vi "PI_Controller.vi"(0 "error":sgl format="%#_13g", 1 "reset? (F)":bool, 2 "Resources":T1, 5 "enable bumpless transfer? (F)":bool, 7 "manual control":T6, 11 "state in":T3, 12 "gains":T4 {"proportional gain" step=0.125}, 13 "output range":T5={"output high (Inf)"=inf, "output low (-Inf)"=-inf}) -> (4 "output":sgl, 6 "error":sgl, 8 "actions":T2, 15 "state out":T3)   [LabVIEW 2017]
uses:
  <vilib>/rvi/Analysis/control/PID/Typedef/niFpgaPID_ManualControl.ctl
  <vilib>/rvi/Analysis/control/PID/Typedef/niFpgaPID_OutputRange.ctl
  <vilib>/rvi/Analysis/control/PID/Typedef/niFpgaPID_PIGains.ctl
  <vilib>/rvi/Analysis/control/PID/Typedef/niFpgaPID_PIState.ctl
  <vilib>/rvi/Analysis/control/PID/Typedef/niFpgaPID_PIActions.ctl
  Multiplier/Multiplier.lvclass
  Adder/Adder.lvclass
  Subtractor/Subtractor.lvclass
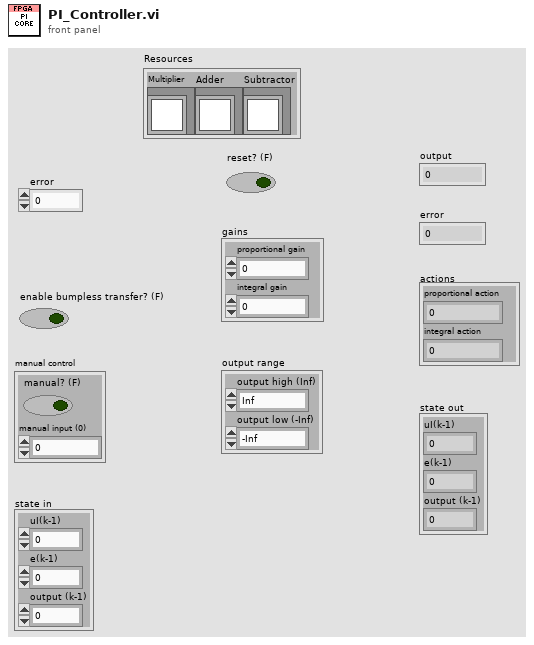
[diagram p1: front panel]
types:
  T1 = cluster{"Multiplier":refnum<class "Multiplier.lvclass">, "Adder":refnum<class "Adder.lvclass">, "Subtractor":refnum<class "Subtractor.lvclass">}
  T2 = typedef "niFpgaPID_PIActions.ctl" = cluster{"proportional action":sgl, "integral action":sgl}
  T3 = typedef "niFpgaPID_PIState.ctl" = cluster{"uI(k-1)":sgl, "e(k-1)":sgl, "output (k-1)":sgl}
  T4 = typedef "niFpgaPID_PIGains.ctl" = cluster{"proportional gain":sgl, "integral gain":sgl}
  T5 = typedef "niFpgaPID_OutputRange.ctl" = cluster{"output high (Inf)":sgl, "output low (-Inf)":sgl}
  T6 = typedef "niFpgaPID_ManualControl.ctl" = cluster{"manual? (F)":bool, "manual input (0)":sgl}
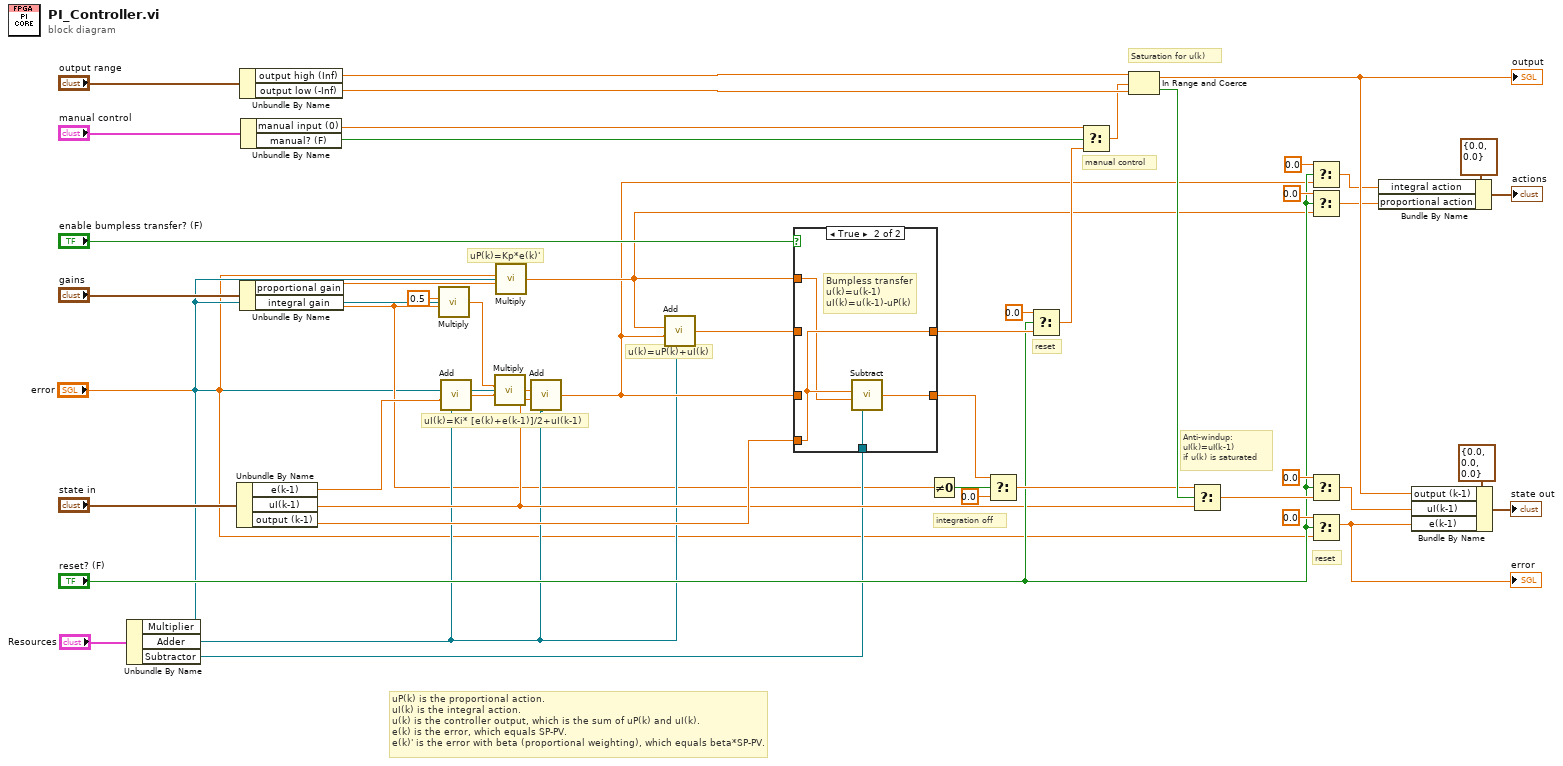
[diagram p0: block diagram]
diagram:
  # "uP(k) is the proportional action.\nuI(k) is the integral action.\nu(k) is the controller output, which is the sum of uP(k) and uI(k).\ne(k) is the error, which equals SP-PV.\ne(k)' is the error with beta (proportional weighting), which equals beta*SP-PV."
  # "integration off"
  # "reset"
  # "manual control"
  # "reset"
  # "Anti-windup:\nuI(k)=uI(k-1) \nif u(k) is saturated"
  # "Saturation for u(k)"
  # "u(k)=uP(k)+uI(k)"
  # "uI(k)=Ki* [e(k)+e(k-1)]/2+uI(k-1)"
  # "uP(k)=Kp*e(k)'"
  n1 = Unbundle By Name("Resources") -> ("Multiplier"=w2:refnum<class "Multiplier.lvclass">, "Adder"=w7:refnum<class "Adder.lvclass">, "Subtractor"=w6:refnum<class "Subtractor.lvclass">)
  n2 = Unbundle By Name("state in") -> ("e(k-1)"=w15:sgl, "uI(k-1)"=w14:sgl, "output (k-1)"=w43:sgl)
  n3 = Unbundle By Name("output range") -> ("output high (Inf)"=w31:sgl, "output low (-Inf)"=w30:sgl)
  n4 = Unbundle By Name("gains") -> ("proportional gain"=w11:sgl, "integral gain"=w4:sgl)
  n5 = Unbundle By Name("manual control") -> ("manual input (0)"=w40:sgl, "manual? (F)"=w39:bool)
  n6 = call-dynamic "Multiply.vi"("x"=sgl 0.5, "y"=w4, "Multiplier"=w2) -> ("x*y"=w5:sgl)  [unwired: 4 in]
  n7 = call-dynamic "Add.vi"("x"="error", "y"=w15, "Adder"=w7) -> ("x+y"=w13:sgl)  [unwired: 4 in]
  n8 = call-dynamic "Multiply.vi"("x"=w5, "y"=w13, "Multiplier"=w2) -> ("x*y"=w12:sgl)  [unwired: 4 in]
  n9 = call-dynamic "Multiply.vi"("x"="error", "y"=w11, "Multiplier"=w2) -> ("x*y"=w10:sgl)  [unwired: 4 in]
  n10 = call-dynamic "Add.vi"("x"=w12, "y"=w14, "Adder"=w7) -> ("x+y"=w9:sgl)  [unwired: 4 in]
  n11 = call-dynamic "Add.vi"("x"=w10, "y"=w9, "Adder"=w7) -> ("x+y"=w8:sgl)  [unwired: 4 in]
  n12 = case shown="True" "enable bumpless transfer? (F)" {
    tunnel: w8 -> [w52 _]
    tunnel: [w52 w56] -> w36
    tunnel: w9 -> [w51 _]
    tunnel: [w51 w54] -> w38
    tunnel: w10 -> [_ w55]
    tunnel: w43 -> [_ w56]
    tunnel: w6 -> [_ w53]
    frame False {
    }
    frame True {
      # "Bumpless transfer\nu(k)=u(k-1)\nuI(k)=u(k-1)-uP(k)"
      n13 = call-dynamic "Subtract.vi"("x"=w56, "y"=w55, "Subtractor"=w53) -> ("x-y"=w54:sgl)  [unwired: 4 in]
    }
  }
  n14 = Not Equal To 0?(x=w4) -> (x != 0?=w42:bool)
  n15 = Select(t=w38, s=w42, f=sgl 0.0) -> (s? t:f=w20:sgl)
  n16 = Select(t=sgl 0.0 ("f"), s="reset? (F)", f=w36) -> (s? t:f=w35:sgl)
  n17 = Select(t=w40, s=w39, f=w35) -> (s? t:f=w29:sgl)
  n18 = In Range and Coerce(upper limit=w31, x=w29, lower limit=w30) -> (coerced(x)=w28:sgl, In Range?=w32:bool)
  "output" <- w28
  n19 = Select(t=w20, s=w32, f=w14) -> (s? t:f=w21:sgl)
  n20 = Select(t=sgl 0.0, s="reset? (F)", f=w9) -> (s? t:f=w24:sgl)
  n21 = Select(t=sgl 0.0, s="reset? (F)", f=w10) -> (s? t:f=w25:sgl)
  n22 = Select(t=sgl 0.0, s="reset? (F)", f=w21) -> (s? t:f=w19:sgl)
  n23 = Select(t=sgl 0.0, s="reset? (F)", f="error") -> (s? t:f=w17:sgl)
  "error" <- w17
  n24 = Bundle By Name(cluster=T2 {"proportional action"=0.0, "integral action"=0.0} ("actions"), "integral action"=w24, "proportional action"=w25) -> (→"actions":T2)
  n25 = Bundle By Name(cluster=T3 {"uI(k-1)"=0.0, "e(k-1)"=0.0, "output (k-1)"=0.0} ("state out"), "output (k-1)"=w28, "uI(k-1)"=w19, "e(k-1)"=w17) -> (→"state out":T3)
